vi "Paint_Tracks_on_Frame-1.vi"(4 "Delete \nOverlay?":bool, 5 "[IN] Number of event":i8, 6 "[IN] Images Array":T1[](array[typedef]), 7 "error IN":errorcluster, 8 "# Frame":u32 max=499, 9 "[IN] #1 Array (X,Y,...)":dbl[][](array[numeric]), 10 "[IN] #1 Processed Image":T1) -> (0 "error OUT":errorcluster, 3 "[OUT] #1 Overlayed Image":T1)   [LabVIEW 2017]
doc: "Drawing of found tracks in frames"
uses:
  <vilib>/vision/Image Controls.llb/IMAQ Image.ctl
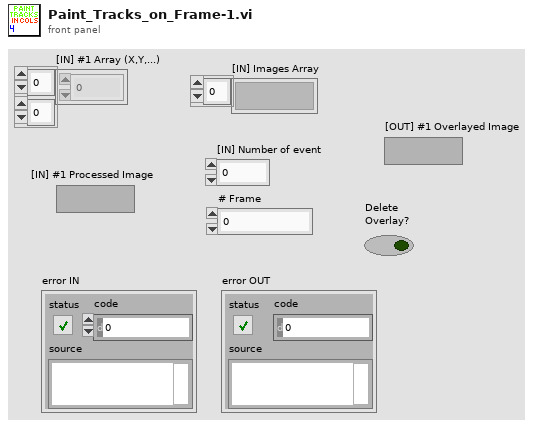
[diagram p1: front panel]
types:
  T1 = typedef "IMAQ Image.ctl" = refnum<image>
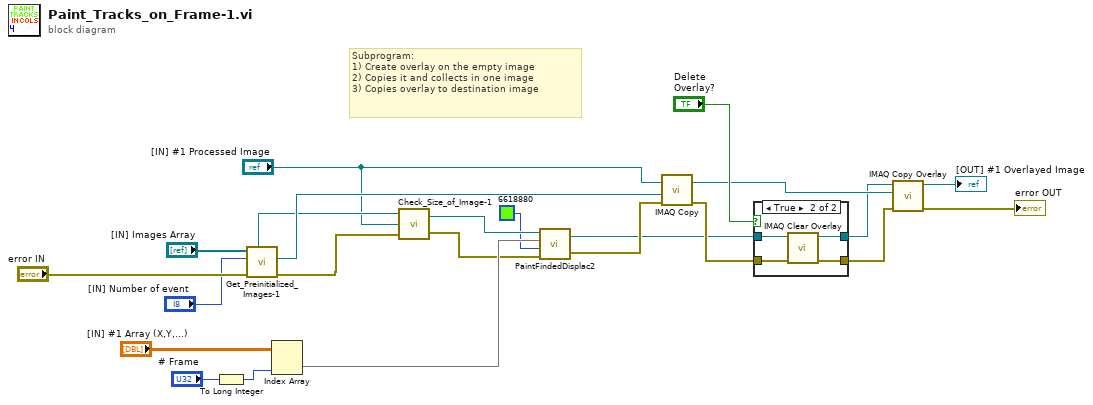
[diagram p0: block diagram]
diagram:
  # "Subprogram:\n1) Create overlay on the empty image\n2) Copies it and collects in one image\n3) Copies overlay to destination image"
  n1 = To Long Integer(number="# Frame") -> (32bit integer=w10:i32)
  n2 = call "Get_Preinitialized_Images-1.vi"("error IN"="error IN", "[IN] Number of event"="[IN] Number of event", "[IN] Images Array"="[IN] Images Array") -> ("error OUT"=w8:errorcluster, "[OUT] Processed Image #1"=w18:T1, "[OUT] Source Image #1"=w17:T1)  [unwired: 1 in, 2 out]
  n3 = Index Array(array="[IN] #1 Array (X,Y,...)", index (col)=w10) -> (element=w14:dbl[])  [unwired: 1 in]
  n4 = call "Check_Size_of_Image-1.vi"("error IN"=w8, "[IN] Source Image"="[IN] #1 Processed Image", "[IN] Image for overlay"=w17) -> ("error OUT"=w12:errorcluster, "[OUT] Image for overlay"=w15:T1)
  n5 = call "PaintFindedDisplac2.vi"("error IN"=w12, "Color of track"=u32 6618880 ("Color"), "Array of Points IN"=w14, "Image IN"=w15) -> ("error OUT"=w11:errorcluster, "Image OUT"=w3:T1)
  n6 = call "IMAQ Copy"("error in (no error)"=w11, "Image Dst"=w18, "Image Src"="[IN] #1 Processed Image") -> ("error out"=w6:errorcluster, "Image Dst Out"=w2:T1)  [unwired: 3 in]
  n7 = case shown="True" "Delete \nOverlay?" {
    tunnel: w3 -> [w25 w29]
    tunnel: [w25 w27] -> w1
    tunnel: w6 -> [w24 w28]
    tunnel: [w24 w26] -> w4
    frame False {
    }
    frame True {
      n8 = call "IMAQ Clear Overlay"("error in (no error)"=w28, "Image"=w29) -> ("error out"=w26:errorcluster, "Image Out"=w27:T1)  [unwired: 8 in]
    }
  }
  n9 = call "IMAQ Copy Overlay"("error in (no error)"=w4, "Image Dst"=w2, "Image Src"=w1) -> ("error out"=→"error OUT":errorcluster, "Image Dst Out"=→"[OUT] #1 Overlayed Image":T1)  [unwired: 7 in]
